vi "infrared_data(SubVI).vi"(6 "input(cm)":dbl) -> (1 "voltage":dbl, 2 "XY Graph":cluster{dbl, dbl}[](graph))   [LabVIEW 2019]
panel:
  out "array of clusters":cluster{dbl, dbl}[](array[cluster])
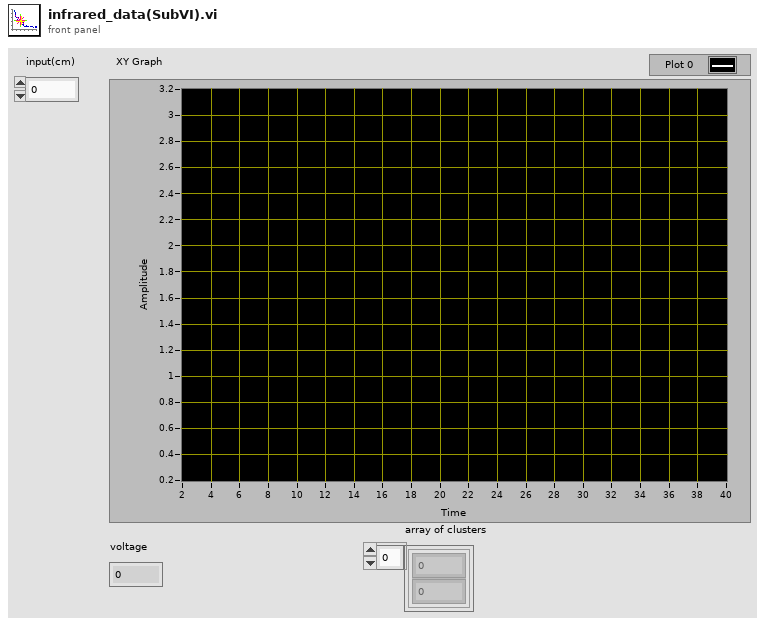
[diagram p1: front panel]
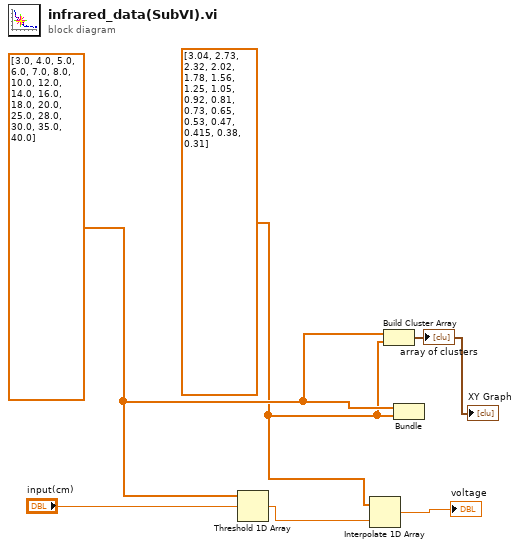
[diagram p0: block diagram]
diagram:
  w2 = dbl[] [3.04, 2.73, 2.32, 2.02, 1.78, 1.56, 1.25, 1.05, 0.92, 0.81, 0.73, 0.65, 0.53, 0.47, 0.415, 0.38, 0.31]
  w3 = dbl[] [3.0, 4.0, 5.0, 6.0, 7.0, 8.0, 10.0, 12.0, 14.0, 16.0, 18.0, 20.0, 25.0, 28.0, 30.0, 35.0, 40.0]
  n1 = Threshold 1D Array(2:"input(cm)", 3:w3) -> (0:w5:dbl)  [unwired: 1 in]
  n2 = Interpolate 1D Array(1:w5, 2:w2) -> (0:→"voltage":dbl)
  n3 = Build Cluster Array(w3, w2) -> (→"XY Graph" →"array of clusters":cluster{dbl, dbl}[])
  n4 = Bundle(w3, w2) -> ()  [unwired: 1 in, 1 out]
